vi "UTIL_Get_Current_Vi_Name v1_0_0.vi"(7 "Path":path) -> (6 "Vi Name":string, 8 "Name Minus Extention":string)   [LabVIEW 2015]
doc: "UTIL_Get_Current_VI_Name.vi\n\nStrips the VI name from path and the extension of .vi\n\nCreated 2006 by\n\nJ. Daren Suntych\nNational Analytics\n970-397-0764"
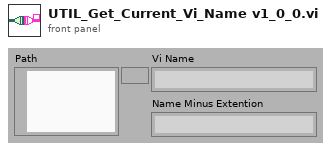
[diagram p1: front panel]
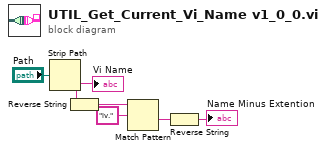
[diagram p0: block diagram]
diagram:
  n1 = Strip Path(path="Path") -> (name=w1:string)  [unwired: 1 out]
  "Vi Name" <- w1
  n2 = Reverse String(1:w1) -> (0:w5:string)
  n3 = Match Pattern(string=w5, regular expression="iv.") -> (after substring=w4:string)  [unwired: 4 out]
  n4 = Reverse String(1:w4) -> (0:→"Name Minus Extention":string)
